vi "convertOldSetlist_toCluster_v5.vi"(0 "HW settings path":path=path "D:/My Documents/NIST (postdoc)/Labview/Data Acquisition/Hardware Control/Hardware/20121128_rbI_default_locked", 1 "Load pre 5.6 Globals?":bool, 5 "Procedure path":path=path "D:/My Documents/NIST (postdoc)/Labview/Data Acquisition/Hardware Control/procedures/201300927_Bzscan_Talbot", 7 "Version Selection":T4=enum."Load DDS 4.10", 11 "error in":errorcluster) -> (4 "Procedure Name":string, 10 "Save Cluster":T2={"Version"="", "Devices"=[], "Select Layout"=0, "Layout:Strings And Values []"=[], "User defined functions"="-- -------------------------------------------------------------------------------------------\n-- The following functions are part of the \"standard load\" of functions and should not be messed with\n-- They are here for reference only.\n-- Please add any user functions above this comment\n-- -------------------------------------------------------------------------------------------\n\n-- Creates a linear ramp from A to B\nfunction LineRamp(f, Initial, Final)\n    return (1-f)*Initial + f*Final;\nend\n\n-- Creates an exponential ramp from A to B\nfunction ExpRamp(t, a, b, tau)\n   return (b - a*exp(tMax / tau) + (a-b)*exp(t/tau))/ ( 1 - exp(tMax / tau) );\nend\n\n-- Creates a sinewave\nfunction SinRamp(t,Offset,A,Freq, Phase)\n    return Offset + A * sin(2*pi*Freq*t + Phase)\nend\n\n-- Creates a blackman pulse\nfunction Blackman(f, Offset, A)\n    return Offset +  A*sqrt(0.5*cos(3.1415*(2*f-1))+0.08*cos(2*pi*(2*f-1))+0.42);\nend\n\n-- Creates a half-gauss ramp\nfunction HalfGaussRamp(t, a, b, Width)\n    local y;\n    y = exp(-(tMax^2)/Width^2);\n    y = (a -  b*y)/(1-y)  +  ((b-a)/(1-y))*exp(-((t-tMax)^2)/Width^2);\n    return y;\nend\n\n-- Creates an \"O'Hara\" ramp from A to B, for dipole evaporation\nfunction EvapRamp(t, a, b, tau)\n   local y;\n  y = log(a/b) / log(1+tMax/tau);\n  y = a * (1+t/tau)^(-y);\n  return y;\nend\n", "VariableManager"=refnum} {"Select Layout" items=["Default"]}, 15 "error out":errorcluster)   [LabVIEW 2013]
uses:
  TypeDefs/Active procedure variables.ctl
  DeviceVIs/DDS/DDS.lvclass
  DeviceVIs/NI Card/NI Card.lvclass
  DeviceVIs/Novatech/Novatech.lvclass
  DeviceVIs/Pulseblaster/Pulseblaster.lvclass
  DeviceVIs/Device/Device.lvclass
  TypeDefs/PreviousVersionSelect.ctl
  TypeDefs/SaveCluster.ctl
  VariableManagerCodes/VariableManager/VariableManager.lvclass
  <vilib>/Utility/miscctls.llb/LVStringsAndValuesArrayTypeDef_I32.ctl
  VariableManagerCodes/API/VariableManagerAPI.lvlib
panel:
  in  "Tab Control":T1(tab)
  out "TempVariableManager":refnum<class "VariableManager.lvclass">
  out "Final PB Master Table":string[][](array[string])
  out "Final NI Device Table":string[][](array[string])
  out "Final Novatech Channel Table":string[][](array[string])
  out "Final DDS Table":string[][](array[string])
  out "DDS Object Array":refnum<class "DDS.lvclass">[](array[class])
  out "NI Card Array":refnum<class "NI Card.lvclass">[](array[class])
  in  "Master PulseBlaster":refnum<class "Pulseblaster.lvclass">
  out "Novatech Object Array":refnum<class "Novatech.lvclass">[](array[class])
  out "Slave PB Array":refnum<class "Pulseblaster.lvclass">[](array[class])
  out "Sequencing Info":T5(array[cluster])
  out "Static Variables":T6[](array[typedef])
  out "Devices":refnum<class "Device.lvclass">[](array[class])
  in  "Select Layout":i32(ring) items=["(On-the-fly)"=-2, "All"=-1, "Legacy"=0]
  out "User defined functions":string
  out "DDS Trig Lines":u16[](array[numeric])
  out "Novatech Trig Lines":u16[](array[numeric])
  out "NI Card Trig Lines":u16[](array[numeric])
  out "Version":string
  out "DDS Devices":T7(array[cluster])
  out "Slave Tables":T8
  out "Master Tables":T8
  out "Novatech Devices":T9(array[cluster])
  out "Novatech Ramps":T10(array[cluster])
  out "NI Cards":T11(array[cluster])
  out "SRS Ramps":T12(array[cluster])
  out "# of DO channels":i32
  out "# of AO channels":i32
  out "# DDS Devices":i32
  out "# Novatech devices":i32
  out "# NI Cards":i32
  out "Length of setlist (lines)":i32
  out "ColHdrs":string[](array[string])
  out "# of AI channels":i32
  # "Debugging:\n\nRight number of rows - YES\nMaster PB - Table = YES\nMaster PB - Hardware?\nDO - Table = Yes \nAO - Table = Yes\nNovatech - ???\nDDS - Table = Yes"
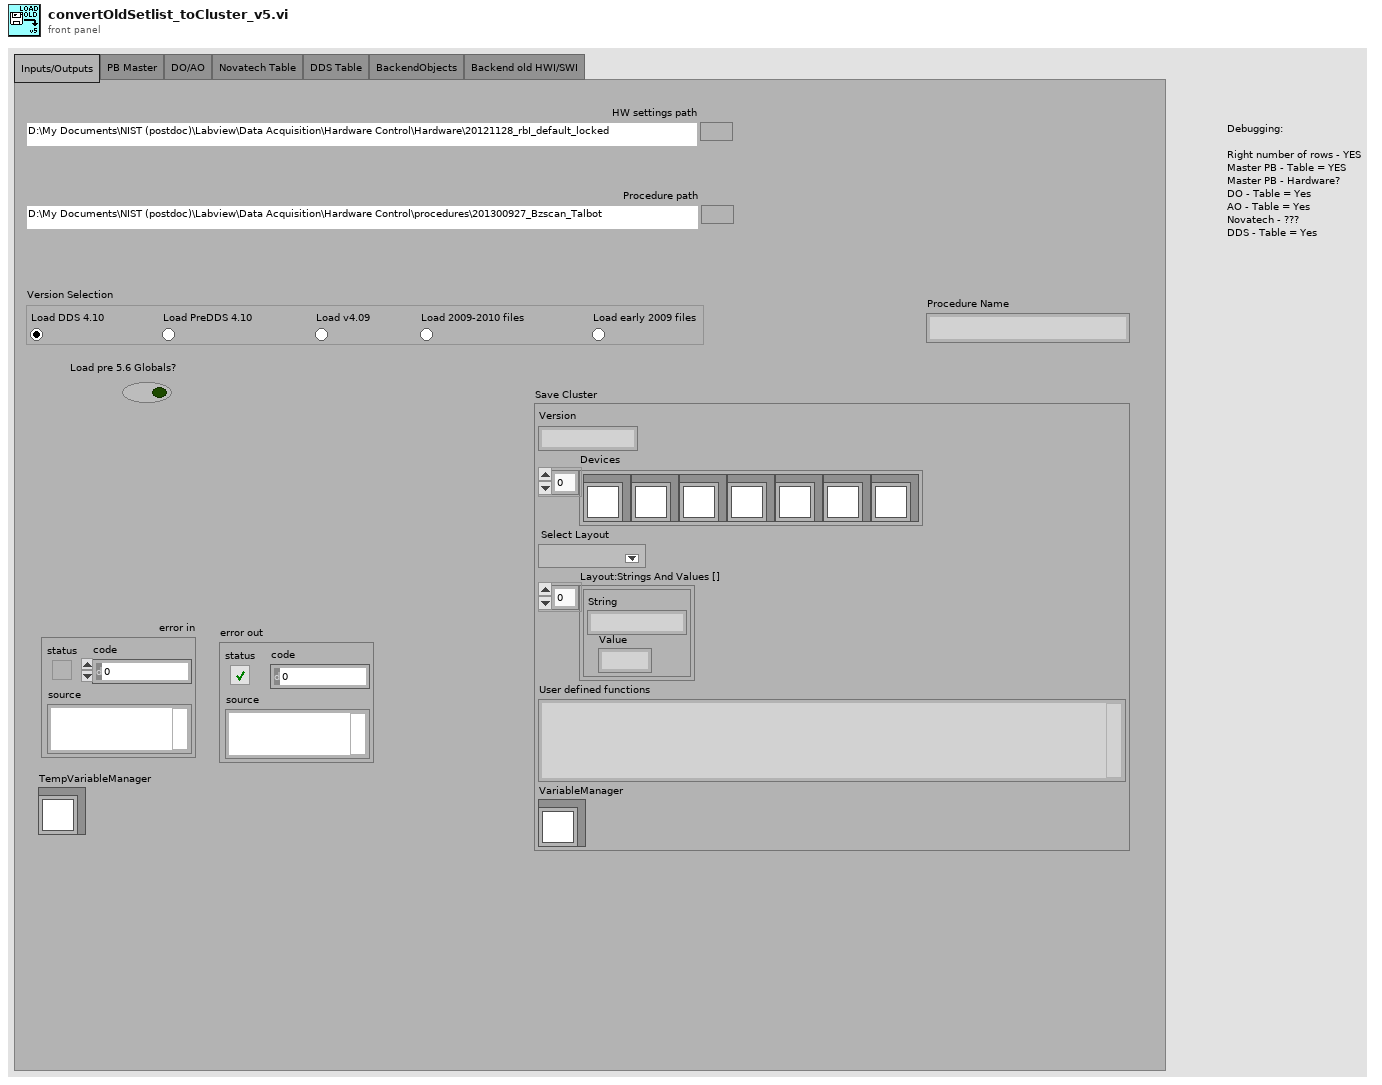
[diagram p1: front panel]
types:
  T1 = enum32{"Inputs/Outputs", "PB Master", "DO/AO", "Novatech Table", "DDS Table", "BackendObjects", "Backend old HWI/SWI"}
  T2 = typedef "SaveCluster.ctl" = cluster{"Version":string, "Devices":refnum<class "Device.lvclass">[], "Select Layout":i32, "Layout:Strings And Values []":T3, "User defined functions":string, "VariableManager":refnum<class "VariableManager.lvclass">}
  T3 = typedef "LVStringsAndValuesArrayTypeDef_I32.ctl" = cluster{"String":string, "Value":i32}[]
  T4 = typedef "PreviousVersionSelect.ctl" = enum32{"Load PreDDS 4.10", "Load early 2009 files", "Load 2009-2010 files", "Load DDS 4.10", "Load v4.09"}
  T5 = cluster{"Start":dbl, "End":dbl, "Sequenced Data":dbl[], "Inform\nIgor?":bool, "Computed Step Size":dbl, "Procedure Variable":string, "Default":dbl, "Steps":i32}[]
  T6 = typedef "Active procedure variables.ctl" = cluster{"Procedure variable":string, "Value":dbl}
  T7 = cluster{"PB Trigger Line":u16, "Sweeps":bool, "Channel Name":string, "Device Description":string, "PB trig / Sequence":bool, "Amp Lock":bool, "SetList Display":bool[], "FPGA Firmware Version":dbl}[]
  T8 = cluster{"Master Staging List":cluster{"Marker":string, "Mode":enum16{"Continue", "Ramp", "Loop", "EndLoop", "Halt"}, "Output Bits":bool[], "Delay (s)":string, "Ramp Step":dbl, "String":string, "Line Number":string}[], "Master DO Table":cluster{"Output Bits":bool[]}[], "Master AO Table":string[][], "Novatech Table":string[][], "DDS Table":string[][]}
  T9 = cluster{"PB Trigger Line":u16, "Serial Port":refnum<visa-resource-name>, "Channel Names":string[], "SetList Display":bool[][]}[]
  T10 = cluster{"Ramp Channels":cluster{"Time":string, "0 Freq. [MHz]":string, "0 Power [dBm]":string, "1 Freq. [MHz]":string, "1 Power [dBm]":string}[], "2 Freq. [MHz]":string, "2 Power [dBm]":string, "3 Freq. [MHz]":string, "3 Power [dBm]":string, "Serial Port":refnum<visa-resource-name>}[]
  T11 = cluster{"AO Channels":refnum<k21>[], "Trigger terminal":tag, "DO Channel":refnum<k21>, "AI Channels":refnum<k21>[], "PB Trigger Line":u16, "Trigger Mirror":tag, "DO lines":i32, "AO Channel Names":string[], "AI Channel Names":string[], "AI Pause Line":tag, "AI Sample Rate":dbl, "SetList Display":bool[]}[]
  T12 = cluster{"lattice ramp":cluster{"dt":string, "formula":string}[], "Output":cluster{"Time Values":dbl[], dbl[]}[], "SRS Selection":enum16{"1550 Vertical", "Bragg Agilent", "Bragg PTS", "Acc. Intensity"}}[]
  T13 = enum32{"Load PreDDS 4.10", "Load early 2009 files", "Load 2009-2010 files", "Load DDS 4.10", "Load v4.09"}
  T14 = cluster{"Master PB Staging List":cluster{"Output Bits":bool[], "Delay (s)":string, "String":string, "Halt?":bool}[], "Slave PB Staging List":cluster{"Output Bits":bool[], "Delay (s)":string, "String":string, "Halt?":bool}[], "Novatech Ramps":cluster{"Ramp Channels":cluster{"Time":string, "0 Freq. [MHz]":string, "0 Power [dBm]":string, "1 Freq. [MHz]":string, "1 Power [dBm]":string}[], "2 Freq. [MHz]":string, "2 Power [dBm]":string, "3 Freq. [MHz]":string, "3 Power [dBm]":string, "Serial Port":refnum<visa-resource-name>}[], "Sequencing Info":cluster{"Start":dbl, "End":dbl, "Sequenced Data":dbl[], "Inform\nIgor?":bool, "Computed Step Size":dbl, "Procedure Variable":string, "Default":dbl, "Steps":i32}[], "SRS Ramps":cluster{"lattice ramp":cluster{"dt":string, "formula":string}[], "Output":cluster{"Time Values":dbl[], dbl[]}[], "SRS Selection":enum16{"1550 Vertical", "Bragg Agilent", "Bragg PTS", "Acc. Intensity"}}[], "Master AO Ramp List":cluster{"Ramp index":u32, "Ramp time [s]":string, "Step size [s]":dbl, "Ramp Array":string[], "Output Bits":bool[]}[], "Slave AO Ramp List":cluster{"Ramp index":u32, "Ramp time [s]":string, "Step size [s]":dbl, "Ramp Array":string[], "Output Bits":bool[]}[], "Master Novatech Ramp List":cluster{"Ramp index":u32, "Ramp time [s]":string, "Step size [s]":dbl, "Data Array":string[]}[], "Static Variables":cluster{"Procedure variable":string, "Value":dbl}[], "DDS Ramp List":cluster{"Ramp index":u32, "Ramp time [s]":string, "Step size [s]":dbl, "Data Array":string[]}[]}
  T15 = cluster{"Master PB Staging List":cluster{"Output Bits":bool[], "Delay (s)":string, "String":string, "Halt?":bool}[], "Slave PB Staging List":cluster{"Output Bits":bool[], "Delay (s)":string, "String":string, "Halt?":bool}[], "Novatech Ramps":cluster{"Ramp Channels":cluster{"Time":string, "0 Freq. [MHz]":string, "0 Power [dBm]":string, "1 Freq. [MHz]":string, "1 Power [dBm]":string}[], "2 Freq. [MHz]":string, "2 Power [dBm]":string, "3 Freq. [MHz]":string, "3 Power [dBm]":string, "Serial Port":refnum<visa-resource-name>}[], "Sequencing Info":cluster{"Start":dbl, "End":dbl, "Sequenced Data":dbl[], "Inform\nIgor?":bool, "Computed Step Size":dbl, "Procedure Variable":string, "Default":dbl, "Steps":i32}[], "SRS Ramps":cluster{"lattice ramp":cluster{"dt":string, "formula":string}[], "Output":cluster{"Time Values":dbl[], dbl[]}[], "SRS Selection":enum16{"1550 Vertical", "Bragg Agilent", "Bragg PTS", "Acc. Intensity"}}[], "Master AO Ramp List":cluster{"Ramp index":u32, "Ramp time [s]":string, "Step size [s]":dbl, "Ramp Array":string[], "Output Bits":bool[]}[], "Slave AO Ramp List":cluster{"Ramp index":u32, "Ramp time [s]":string, "Step size [s]":dbl, "Ramp Array":string[], "Output Bits":bool[]}[], "Master Novatech Ramp List":cluster{"Ramp index":u32, "Ramp time [s]":string, "Step size [s]":dbl, "Data Array":string[]}[], "Static Variables":T6[], "DDS Ramp List":cluster{"Ramp index":u32, "Ramp time [s]":string, "Step size [s]":dbl, "Data Array":string[]}[]}
  T16 = cluster{"User defined functions":string, "Master AO Channels":cluster{"AO Channels":refnum<k21>[], "Trigger terminal":tag, "DO Channel":refnum<k21>, "AI Channels":refnum<k21>[], "PB Trigger Line":u16, "Trigger Mirror":tag, "DO lines":i32, "AO Channel Names":string[], "AI Channel Names":string[], "AI Pause Line":tag, "AI Sample Rate":dbl, "SetList Display":bool[]}[], "Novatech Devices":cluster{"PB Trigger Line":u16, "Serial Port":refnum<visa-resource-name>, "Channel Names":string[], "SetList Display":bool[][]}[], "DDS Devices":cluster{"PB Trigger Line":u16, "Sweeps":bool, "Channel Name":string, "Device Description":string, "PB trig / Sequence":bool, "Amp Lock":bool, "SetList Display":bool[], "FPGA Firmware Version":dbl}[]}
  T17 = cluster{"Output Bits":bool[], "Delay (s)":string, "String":string, "Halt?":bool}[]
  T18 = cluster{"Ramp index":u32, "Ramp time [s]":string, "Step size [s]":dbl, "Ramp Array":string[], "Output Bits":bool[]}[]
  T19 = cluster{"Ramp index":u32, "Ramp time [s]":string, "Step size [s]":dbl, "Data Array":string[]}[]
  T20 = cluster{"Marker":string, "Mode":enum16{"Continue", "Ramp", "Loop", "EndLoop", "Halt"}, "Output Bits":bool[], "Delay (s)":string, "Ramp Step":dbl, "String":string, "Line Number":string}[]
  T21 = enum16{"Continue", "Ramp", "Loop", "EndLoop", "Halt"}
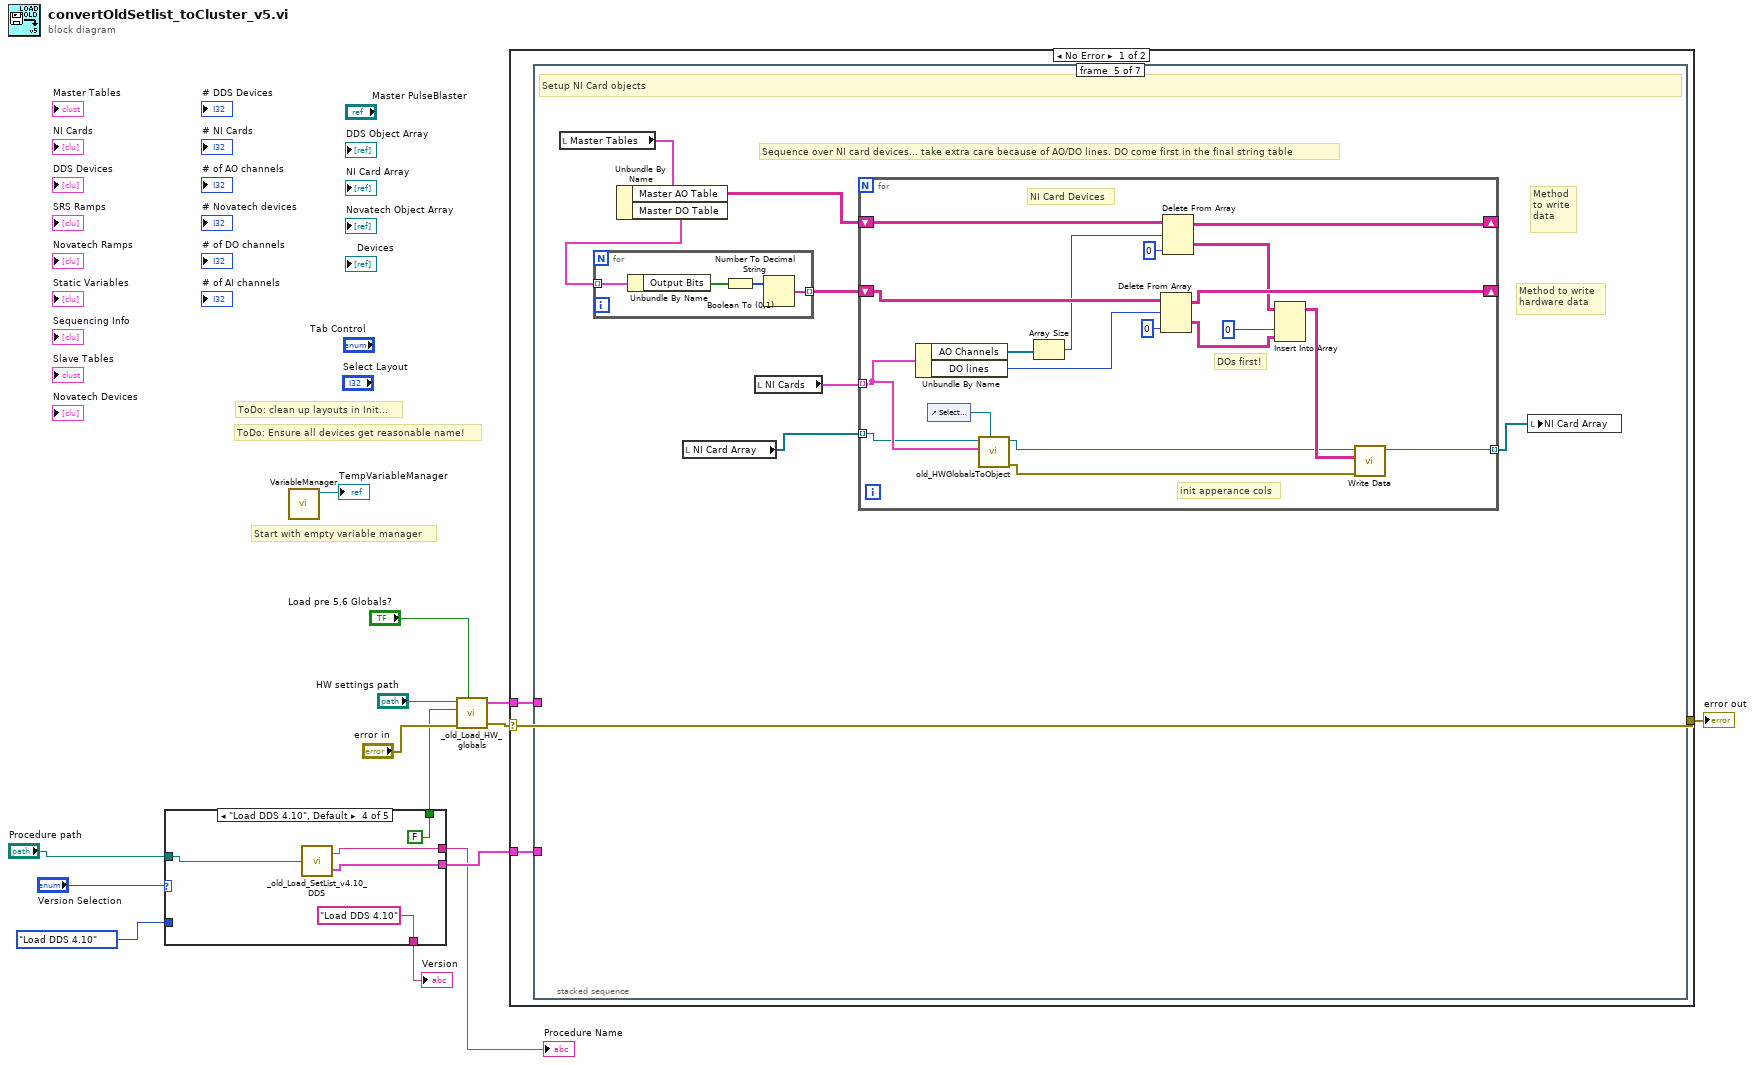
[diagram p0: block diagram]
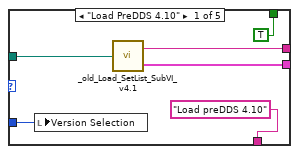
[diagram p2: hidden frame]
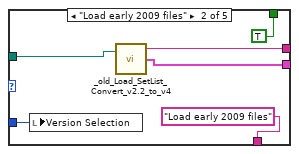
[diagram p3: hidden frame]
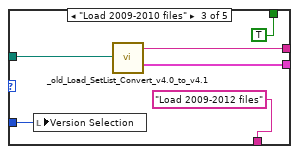
[diagram p4: hidden frame]
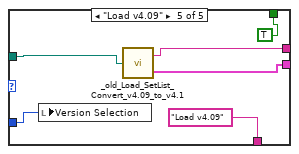
[diagram p5: hidden frame]
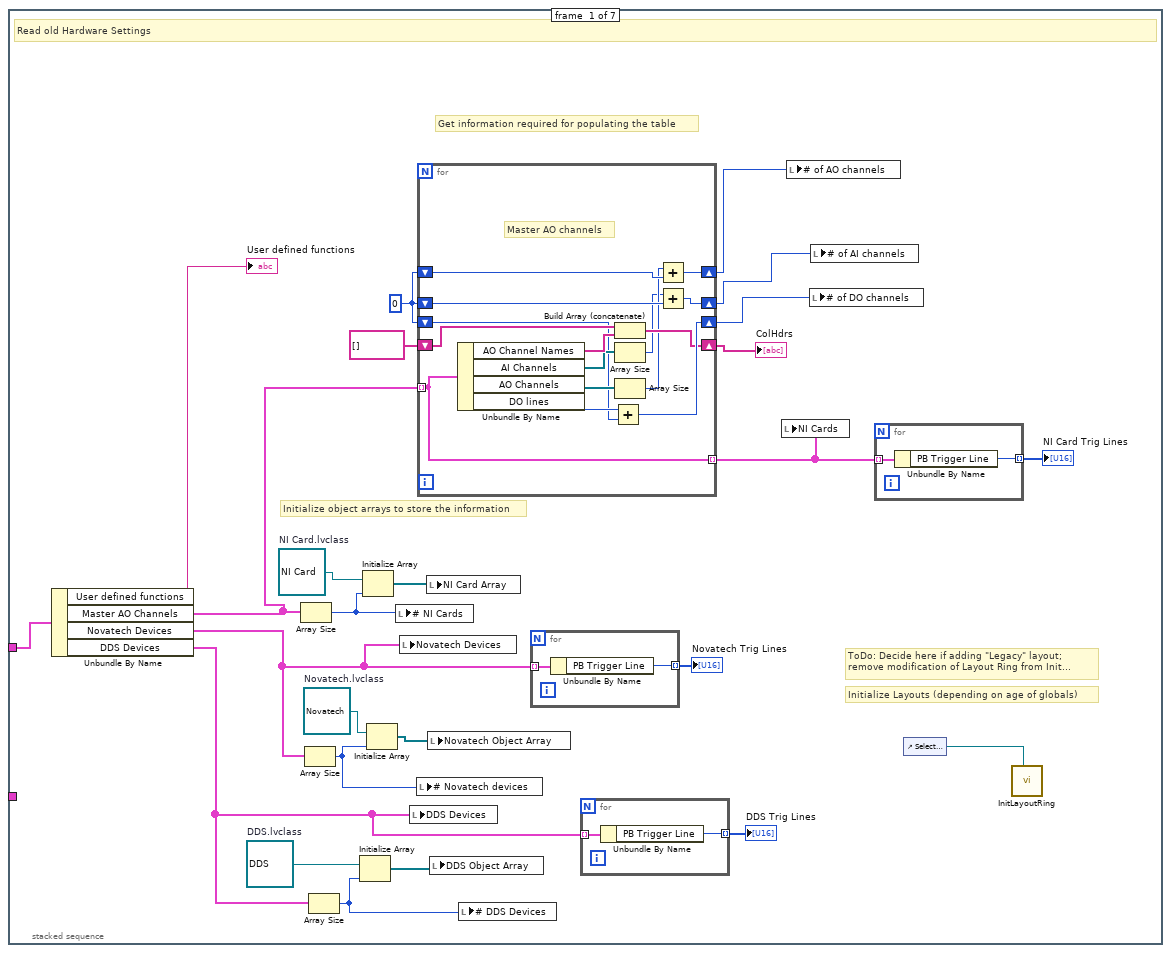
[diagram p6: hidden frame]
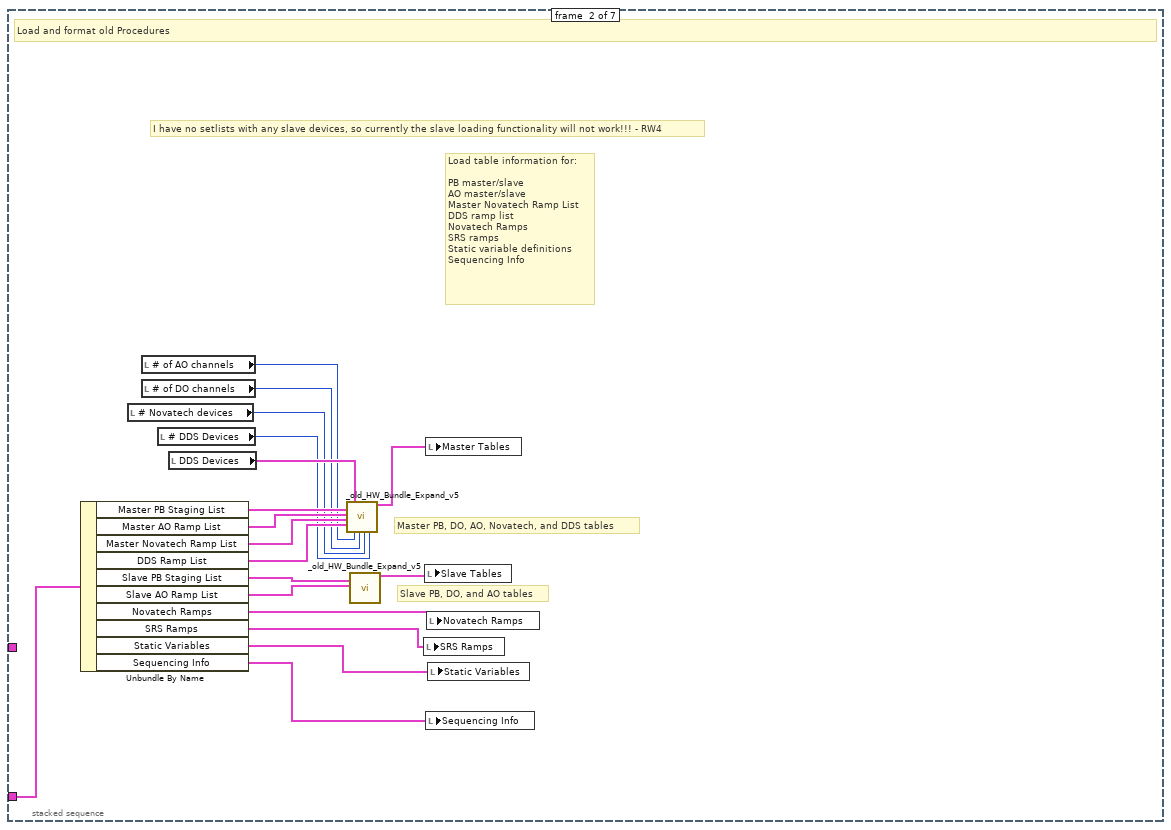
[diagram p7: hidden frame]
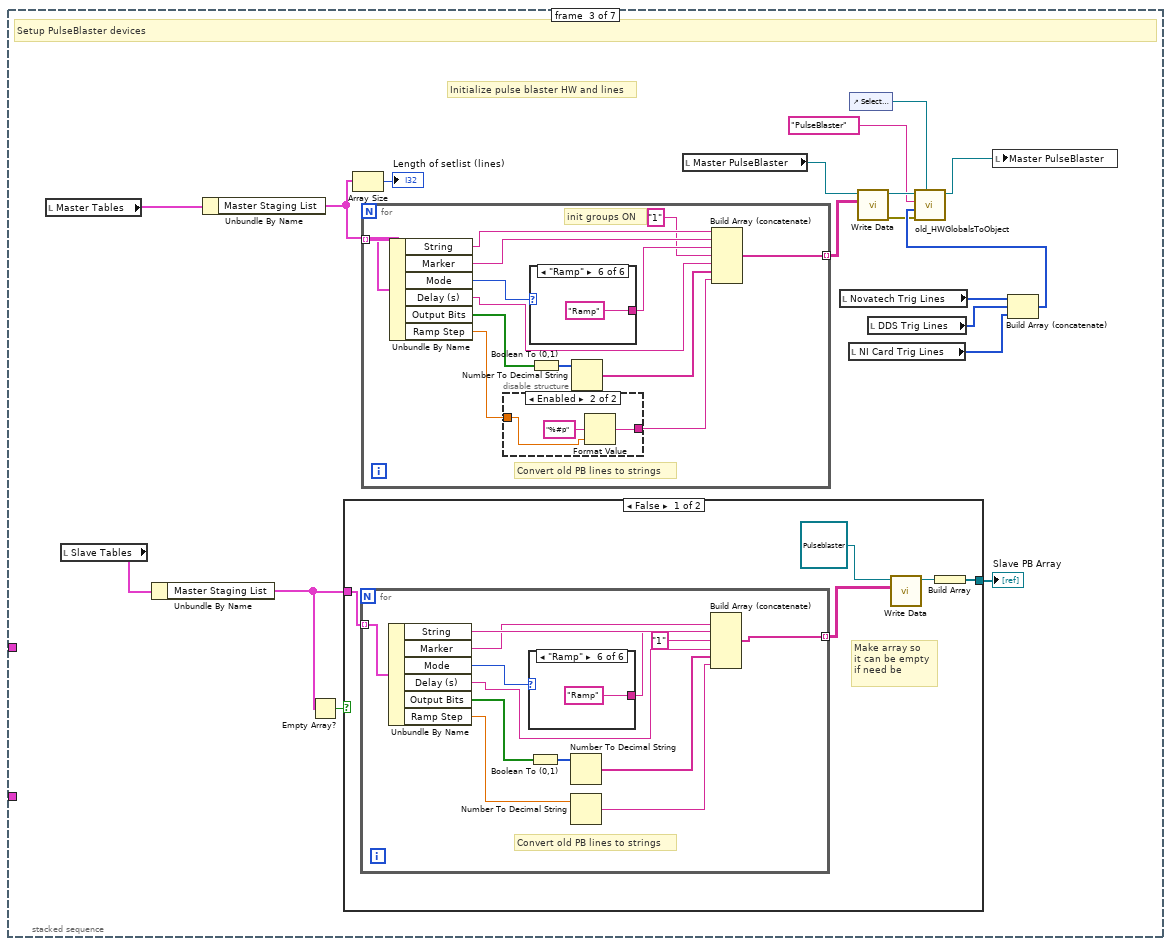
[diagram p8: hidden frame]
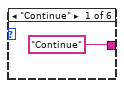
[diagram p9: hidden frame]
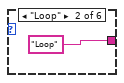
[diagram p10: hidden frame]
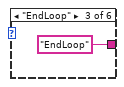
[diagram p11: hidden frame]
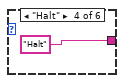
[diagram p12: hidden frame]
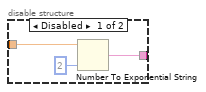
[diagram p15: hidden frame]
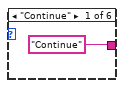
[diagram p16: hidden frame]
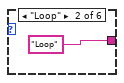
[diagram p17: hidden frame]
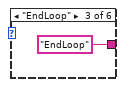
[diagram p18: hidden frame]
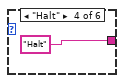
[diagram p19: hidden frame]
diagram:
  # "Start with empty variable manager"
  # "ToDo: Ensure all devices get reasonable name!"
  # "ToDo: clean up layouts in Init..."
  n1 = case shown="\"Load DDS 4.10\", Default" "Version Selection" {
    tunnel: [w20 w25 w32 w36 w40] -> w6
    tunnel: "Procedure path" -> [w19 w26 w30 w37 w41]
    tunnel: [w18 w24 w31 w35 w39] -> w7
    tunnel: T13."Load DDS 4.10" ("Version Selection") -> [w17 w23 w29 _ w43]
    tunnel: [TRUE TRUE TRUE FALSE TRUE] -> w4
    tunnel: ["Load preDDS 4.10" "Load early 2009 files" "Load 2009-2012 files" "Load DDS 4.10" "Load v4.09"] -> w2
    frame "Load PreDDS 4.10" {
      n2 = local write "Version Selection"(w17) -> ()
      n3 = call "_old_Load_SetList_SubVI_v4.1.vi"("Path"=w19) -> ("Procedure Name"=w20:string, "Paramaters"=w18:T14)
    }
    frame "Load early 2009 files" {
      n4 = local write "Version Selection"(w23) -> ()
      n5 = call "_old_Load_SetList_Convert_v2.2_to_v4.vi"("Path"=w26) -> ("Procedure Name"=w25:string, "Paramaters"=w24:T14)  [unwired: 1 in, 1 out]
    }
    frame "Load 2009-2010 files" {
      n6 = local write "Version Selection"(w29) -> ()
      n7 = call "_old_Load_SetList_Convert_v4.0_to_v4.1.vi"("Path"=w30) -> ("Procedure Name"=w32:string, "Paramaters"=w31:T14)
    }
    frame "Load DDS 4.10", Default {
      n8 = call "_old_Load_SetList_v4.10_DDS.vi"("Path"=w37) -> ("Procedure Name"=w36:string, "Paramaters"=w35:T15)
    }
    frame "Load v4.09" {
      n9 = local write "Version Selection"(w43) -> ()
      n10 = call "_old_Load_SetList_Convert_v4.09_to_v4.1.vi"("Path"=w41) -> ("Procedure Name"=w40:string, "Paramaters"=w39:T14)
    }
  }
  "Procedure Name" <- w6
  "Version" <- w2
  n11 = call "VariableManager.vi"() -> ("VariableManager"=→"TempVariableManager":refnum<class "VariableManager.lvclass">)  [unwired: 11 in]
  n12 = call "_old_Load_HW_globals.vi"("HW settings path"="HW settings path", "Load pre 5.6 Globals?"="Load pre 5.6 Globals?", "Pre 4.1 HWGlobals?"=w4, "error in"="error in") -> ("Loaded Procedure Data"=w14:T16, "error out"=w3:errorcluster)  [unwired: 2 in, 1 out]
  n13 = case shown="No Error" w3 {
    selector: w3 -> [w44 w315]
    tunnel: w7 -> [w45 _]
    tunnel: w14 -> [w46 _]
    tunnel: [w44 w315] -> w10
    frame No Error {
      n14 = stacked-sequence {
        tunnel: w46 -> [w71 _ _ _ _ _ _]
        tunnel: w45 -> [_ w110 _ _ _ _ _]
        frame #0 {
          w61 = refnum<class "Novatech.lvclass"> refnum  # Novatech.lvclass
          w62 = refnum<class "NI Card.lvclass"> refnum  # NI Card.lvclass
          w63 = refnum<class "DDS.lvclass"> refnum  # DDS.lvclass
          w68 = 0
          # "ToDo: Decide here if adding \"Legacy\" layout;\nremove modification of Layout Ring from Init..."
          # "Initialize Layouts (depending on age of globals)"
          # "Initialize object arrays to store the information"
          # "Get information required for populating the table"
          # "Read old Hardware Settings"
          n15 = Unbundle By Name(w71) -> ("User defined functions"=→"User defined functions":string, "Master AO Channels"=w67:T11, "Novatech Devices"=w54:T9, "DDS Devices"=w52:T7)
          n16 = Array Size(array=w67) -> (size(s)=w60:i32)
          n17 = Array Size(array=w54) -> (size(s)=w57:i32)
          n18 = Array Size(array=w52) -> (size(s)=w58:i32)
          n19 = Initialize Array(w63, w58) -> (w47:refnum<class "DDS.lvclass">[])
          n20 = Initialize Array(w62, w60) -> (w49:refnum<class "NI Card.lvclass">[])
          n21 = Initialize Array(w61, w57) -> (w48:refnum<class "Novatech.lvclass">[])
          n22 = local write "# NI Cards"(w60) -> ()
          n23 = local write "Novatech Devices"(w54) -> ()
          n24 = local write "DDS Devices"(w52) -> ()
          n25 = local write "# Novatech devices"(w57) -> ()
          n26 = for {
            tunnel: w67 -> [w81] mode=indexing
            shift-right: [w90] -> w65
            shift-left: w68 -> [w79]
            shift-right: [w89] -> w64
            shift-left: w68 -> [w91]
            shift-right: [w88] -> w66
            shift-left: w68 -> [w92]
            shift-right: [w84] -> w69
            shift-left: string[] [] ("initialized array") -> [w85]
            tunnel: [w81] -> w56 mode=indexing
            # "Master AO channels"
            n27 = Unbundle By Name(w81) -> ("AO Channel Names"=w86:string[], "AI Channels"=w83:refnum<k21>[], "AO Channels"=w82:refnum<k21>[], "DO lines"=w87:i32)
            n28 = Add(x=w87, y=w79) -> (x+y=w90:i32)
            n29 = Build Array (concatenate)(w85, w86) -> (w84:string[])
            n30 = Array Size(array=w83) -> (size(s)=w78:i32)
            n31 = Array Size(array=w82) -> (size(s)=w80:i32)
            n32 = Add(x=w80, y=w92) -> (x+y=w88:i32)
            n33 = Add(x=w78, y=w91) -> (x+y=w89:i32)
          }
          "ColHdrs" <- w69
          n34 = local write "NI Card Array"(w49) -> ()
          n35 = local write "Novatech Object Array"(w48) -> ()
          n36 = local write "DDS Object Array"(w47) -> ()
          n37 = local write "# DDS Devices"(w58) -> ()
          n38 = for {
            tunnel: w54 -> [w75] mode=indexing
            tunnel: [w74] -> w53 mode=indexing
            n39 = Unbundle By Name(w75) -> ("PB Trigger Line"=w74:u16)
          }
          "Novatech Trig Lines" <- w53
          n40 = for {
            tunnel: w52 -> [w73] mode=indexing
            tunnel: [w72] -> w51 mode=indexing
            n41 = Unbundle By Name(w73) -> ("PB Trigger Line"=w72:u16)
          }
          "DDS Trig Lines" <- w51
          n42 = local write "NI Cards"(w56) -> ()
          n43 = local write "# of AO channels"(w66) -> ()
          n44 = local write "# of DO channels"(w65) -> ()
          n45 = local write "# of AI channels"(w64) -> ()
          n46 = for {
            tunnel: w56 -> [w77] mode=indexing
            tunnel: [w76] -> w55 mode=indexing
            n47 = Unbundle By Name(w77) -> ("PB Trigger Line"=w76:u16)
          }
          "NI Card Trig Lines" <- w55
          n48 = control-ref of="Select Layout"() -> (w50:refnum<vi>)
          n49 = call "InitLayoutRing.vi"("Layouts Ring Refnum"=w50) -> ()  [unwired: 10 in, 1 out]
        }
        frame #1 {
          # "I have no setlists with any slave devices, so currently the slave loading functionality will not work!!! - RW4"
          # "Load table information for:\n\nPB master/slave\nAO master/slave\nMaster Novatech Ramp List\nDDS ramp list\nNovatech Ramps\nSRS ramps\nStatic variable definitions\nSequencing Info"
          # "Slave PB, DO, and AO tables"
          # "Master PB, DO, AO, Novatech, and DDS tables"
          # "Load and format old Procedures"
          n50 = Unbundle By Name(w110) -> ("Master PB Staging List"=w109:T17, "Master AO Ramp List"=w108:T18, "Master Novatech Ramp List"=w107:T19, "DDS Ramp List"=w106:T19, "Slave PB Staging List"=w104:T17, "Slave AO Ramp List"=w103:T18, "Novatech Ramps"=w101:T10, "SRS Ramps"=w102:T12, "Static Variables"=w99:T6[], "Sequencing Info"=w100:T5)
          n51 = local read "# Novatech devices"() -> (w94:i32)
          n52 = local read "# of AO channels"() -> (w96:i32)
          n53 = local read "# of DO channels"() -> (w95:i32)
          n54 = local read "# DDS Devices"() -> (w93:i32)
          n55 = local read "DDS Devices"() -> (w105:T7)
          n56 = call "_old_HW_Bundle_Expand_v5.vi"("PB Staging List"=w109, "AO Ramp List"=w108, "Novatech Ramp List"=w107, "DDS Ramp List"=w106, "DDS Devices"=w105, "Number of AO channels"=w96, "Number of DO channels"=w95, "Number of Novatech channels"=w94, "Number of DDS channels"=w93) -> ("Master Tables"=w98:T8)  [unwired: 10 in]
          n57 = call "_old_HW_Bundle_Expand_v5.vi"("PB Staging List"=w104, "AO Ramp List"=w103) -> ("Master Tables"=w97:T8)  [unwired: 17 in]
          n58 = local write "SRS Ramps"(w102) -> ()
          n59 = local write "Slave Tables"(w97) -> ()
          n60 = local write "Master Tables"(w98) -> ()
          n61 = local write "Sequencing Info"(w100) -> ()
          n62 = local write "Novatech Ramps"(w101) -> ()
          n63 = local write "Static Variables"(w99) -> ()
        }
        frame #2 {
          # "Initialize pulse blaster HW and lines"
          # "Setup PulseBlaster devices"
          n64 = local read "Master Tables"() -> (w128:T8)
          n65 = local read "Slave Tables"() -> (w123:T8)
          n66 = Unbundle By Name(w123) -> ("Master Staging List"=w122:T20)
          n67 = Unbundle By Name(w128) -> ("Master Staging List"=w126:T20)
          n68 = Empty Array?(array=w122) -> (empty?=w121:bool)
          n69 = case shown="False" w121 {
            tunnel: w122 -> [w132 _]
            tunnel: [w130 _] -> w111
            frame False {
              # "Make array so\nit can be empty\nif need be"
              n70 = for {
                tunnel: w132 -> [w146] mode=indexing
                tunnel: [w138] -> w133 mode=indexing
                # "Convert old PB lines to strings"
                n71 = Unbundle By Name(w146) -> ("String"=w145:string, "Marker"=w144:string, "Mode"=w143:T21, "Delay (s)"=w135:string, "Output Bits"=w140:bool[], "Ramp Step"=w141:dbl)
                n72 = case shown="\"Ramp\"" w143 {
                  tunnel: ["Continue" "Loop" "EndLoop" "Halt" _ "Ramp"] -> w142
                  frame "Continue" {
                  }
                  frame "Loop" {
                  }
                  frame "EndLoop" {
                  }
                  frame "Halt" {
                  }
                  frame Default {
                  }
                  frame "Ramp" {
                  }
                }
                n73 = Boolean To (0,1)(Boolean=w140) -> (0, 1=w139:i16[])
                n74 = Number To Decimal String(number=w139) -> (decimal integer string=w136:string[])  [unwired: 1 in]
                n75 = Number To Decimal String(number=w141) -> (decimal integer string=w137:string)  [unwired: 1 in]
                n76 = Build Array (concatenate)(w145, w144, w142, "1" ("element"), w135, w136, w137) -> (w138:string[])
              }
              n77 = call-dynamic "Write Data.vi"("Data"=w133, "Device in"=refnum<class "Pulseblaster.lvclass"> refnum ("Master PulseBlaster")) -> ("Device Out"=w131:refnum<class "Pulseblaster.lvclass">)  [unwired: 8 in, 1 out]
              n78 = Build Array(w131) -> (w130:refnum<class "Pulseblaster.lvclass">[])
            }
            frame True {
              # "No Slave PB"
            }
          }
          "Slave PB Array" <- w111
          n79 = Array Size(array=w126) -> (size(s)=→"Length of setlist (lines)":i32)
          n80 = for {
            tunnel: w126 -> [w164] mode=indexing
            tunnel: [w157] -> w125 mode=indexing
            # "init groups ON"
            # "Convert old PB lines to strings"
            n81 = Unbundle By Name(w164) -> ("String"=w163:string, "Marker"=w162:string, "Mode"=w161:T21, "Delay (s)"=w155:string, "Output Bits"=w159:bool[], "Ramp Step"=w152:dbl)
            n82 = disable-structure shown="Enabled" {
              disable-tunnel: [w167 w169] -> w153
              disable-tunnel: w152 -> [w166 w168]
              frame Disabled {
                n83 = Number To Exponential String(number=w166, precision (6)=i16 2) -> (E-format string=w167:string)  [unwired: 2 in]
              }
              frame Enabled {
                n84 = Format Value(format string="%#p", value (0)=w168) -> (output string=w169:string)  [unwired: 1 in]
              }
            }
            n85 = case shown="\"Ramp\"" w161 {
              tunnel: ["Continue" "Loop" "EndLoop" "Halt" _ "Ramp"] -> w160
              frame "Continue" {
              }
              frame "Loop" {
              }
              frame "EndLoop" {
              }
              frame "Halt" {
              }
              frame Default {
              }
              frame "Ramp" {
              }
            }
            n86 = Boolean To (0,1)(Boolean=w159) -> (0, 1=w158:i16[])
            n87 = Number To Decimal String(number=w158) -> (decimal integer string=w156:string[])  [unwired: 1 in]
            n88 = Build Array (concatenate)(w163, w162, w160, "1" ("element"), w155, w156, w153) -> (w157:string[])
          }
          n89 = local read "Master PulseBlaster"() -> (w124:refnum<class "Pulseblaster.lvclass">)
          n90 = local read "Novatech Trig Lines"() -> (w117:u16[])
          n91 = local read "NI Card Trig Lines"() -> (w115:u16[])
          n92 = control-ref of="Select Layout"() -> (w112:refnum<vi>)
          n93 = call-dynamic "Write Data.vi"("Data"=w125, "Device in"=w124) -> ("error out"=w113:errorcluster, "Device Out"=w120:refnum<class "Pulseblaster.lvclass">)  [unwired: 8 in]
          n94 = local read "DDS Trig Lines"() -> (w116:u16[])
          n95 = Build Array (concatenate)(w117, w116, w115) -> (w114:u16[])
          n96 = call "old_HWGlobalsToObject.vi"("Select Layout"=w112, "error in (no error)"=w113, "Trigger Lines"=w114, "Name"="PulseBlaster", "Pulseblaster in"=w120) -> ("Pulseblaster out"=w119:refnum<class "Pulseblaster.lvclass">)  [unwired: 5 in, 1 out]
          n97 = local write "Master PulseBlaster"(w119) -> ()
        }
        frame #3 {
          # "Sequence over old master tables\nGrab individual software image table that corresponds to each device"
          # "Setup Novatech and DDS devices"
          n98 = local read "Master Tables"() -> (w180:T8)
          n99 = local read "Novatech Object Array"() -> (w178:refnum<class "Novatech.lvclass">[])
          n100 = Unbundle By Name(w180) -> ("DDS Table"=w183:string[][])
          n101 = Unbundle By Name(w180) -> ("Novatech Table"=w182:string[][])
          n102 = local read "Novatech Devices"() -> (w181:T9)
          n103 = local read "DDS Object Array"() -> (w179:refnum<class "DDS.lvclass">[])
          n104 = local read "DDS Devices"() -> (w184:T7)
          n105 = for {
            tunnel: w179 -> [w201] mode=indexing
            tunnel: w184 -> [w199] mode=indexing
            shift-right: [w202] -> _
            shift-left: w183 -> [w206]
            tunnel: [w203] -> w176 mode=indexing
            # "DDS Devices"
            n106 = control-ref of="Select Layout"() -> (w197:refnum<vi>)
            n107 = Unbundle By Name(w199) -> ("Sweeps"=w207:bool)
            n108 = call "old_HWGlobalsToObject.vi"("Select Layout"=w197, "DDS Device"=w199, "DDS in"=w201) -> ("error out"=w196:errorcluster, "DDS out"=w200:refnum<class "DDS.lvclass">)  [unwired: 7 in]
            n109 = case shown="False" w207 {
              tunnel: [3 5] -> w204
              frame False {
              }
              frame True {
              }
            }
            n110 = Delete From Array(array=w206, length=w204, index (col)=0 ("disabled index (col)")) -> (deleted portion=w198:string[][], array with subset deleted=w202:string[][])  [unwired: 1 in]
            n111 = call-dynamic "Write Data.vi"("error in (no error)"=w196, "Data"=w198, "Device in"=w200) -> ("Device Out"=w203:refnum<class "DDS.lvclass">)  [unwired: 7 in, 1 out]
          }
          n112 = for {
            tunnel: w178 -> [w189] mode=indexing
            tunnel: w181 -> [w187] mode=indexing
            shift-right: [w194] -> _
            shift-left: w182 -> [w195]
            tunnel: [w191] -> w177 mode=indexing
            # "Novatech Devices"
            n113 = control-ref of="Select Layout"() -> (w186:refnum<vi>)
            n114 = Delete From Array(array=w195, length=12, index (col)=0 ("disabled index (col)")) -> (deleted portion=w190:string[][], array with subset deleted=w194:string[][])  [unwired: 1 in]
            n115 = call "old_HWGlobalsToObject.vi"("Select Layout"=w186, "Novatech Channel"=w187, "Novatech in"=w189) -> ("error out"=w185:errorcluster, "Novatech out"=w188:refnum<class "Novatech.lvclass">)  [unwired: 7 in]
            n116 = call-dynamic "Write Data.vi"("error in (no error)"=w185, "Data"=w190, "Device in"=w188) -> ("Device Out"=w191:refnum<class "Novatech.lvclass">)  [unwired: 7 in, 1 out]
          }
          n117 = local write "Novatech Object Array"(w177) -> ()
          n118 = local write "DDS Object Array"(w176) -> ()
        }
        frame #4 {
          # "Sequence over NI card devices... take extra care because of AO/DO lines. DO come first in the final string table"
          # "Method to write\nhardware data"
          # "Method\nto write\ndata"
          # "Setup NI Card objects"
          n119 = local read "Master Tables"() -> (w215:T8)
          n120 = Unbundle By Name(w215) -> ("Master AO Table"=w214:string[][], "Master DO Table"=w213:cluster{"Output Bits":bool[]}[])
          n121 = for {
            tunnel: [w218] -> w212 mode=indexing
            tunnel: w213 -> [w217] mode=indexing
            n122 = Unbundle By Name(w217) -> ("Output Bits"=w220:bool[])
            n123 = Boolean To (0,1)(Boolean=w220) -> (0, 1=w219:i16[])
            n124 = Number To Decimal String(number=w219) -> (decimal integer string=w218:string[])  [unwired: 1 in]
          }
          n125 = local read "NI Card Array"() -> (w211:refnum<class "NI Card.lvclass">[])
          n126 = local read "NI Cards"() -> (w216:T11)
          n127 = for {
            shift-right: [w233] -> _
            shift-left: w214 -> [w239]
            tunnel: w216 -> [w229] mode=indexing
            shift-right: [w234] -> _
            shift-left: w212 -> [w236]
            tunnel: [w230] -> w210 mode=indexing
            tunnel: w211 -> [w228] mode=indexing
            # "init apperance cols"
            # "DOs first!"
            # "NI Card Devices"
            n128 = Unbundle By Name(w229) -> ("AO Channels"=w235:refnum<k21>[], "DO lines"=w224:i32)
            n129 = control-ref of="Select Layout"() -> (w221:refnum<vi>)
            n130 = call "old_HWGlobalsToObject.vi"("Select Layout"=w221, "Master AO Channel"=w229, "NI Card in"=w228) -> ("error out"=w222:errorcluster, "NI Card out"=w223:refnum<class "NI Card.lvclass">)  [unwired: 7 in]
            n131 = Array Size(array=w235) -> (size(s)=w225:i32)
            n132 = Delete From Array(array=w236, length=w224, index (col)=0 ("disabled index (col)")) -> (deleted portion=w226:string[][], array with subset deleted=w234:string[][])  [unwired: 1 in]
            n133 = Delete From Array(array=w239, length=w225, index (col)=0 ("disabled index (col)")) -> (deleted portion=w227:string[][], array with subset deleted=w233:string[][])  [unwired: 1 in]
            n134 = Insert Into Array(array=w227, index (col)=0 ("disabled index (col)"), new element=w226) -> (w231:string[][])  [unwired: 1 in]
            n135 = call-dynamic "Write Data.vi"("error in (no error)"=w222, "Data"=w231, "Device in"=w223) -> ("Device Out"=w230:refnum<class "NI Card.lvclass">)  [unwired: 7 in, 1 out]
          }
          n136 = local write "NI Card Array"(w210) -> ()
        }
        frame #5 {
          # "Store final device object array"
          # "Build device array; Device tables for testing"
          n137 = local read "Master PulseBlaster"() -> (w254:refnum<class "Pulseblaster.lvclass">)
          n138 = local read "Novatech Object Array"() -> (w240:refnum<class "Novatech.lvclass">[])
          n139 = local read "DDS Object Array"() -> (w242:refnum<class "DDS.lvclass">[])
          n140 = local read "NI Card Array"() -> (w241:refnum<class "NI Card.lvclass">[])
          n141 = Build Array(w254) -> (w253:refnum<class "Pulseblaster.lvclass">[])
          n142 = Insert Into Array(array=refnum<class "Device.lvclass">[] [] ("Devices 2"), new element #1=w253, new element #2=w241, new element #3=w240, new element #4=w242) -> (w243:refnum<class "Device.lvclass">[])  [unwired: 1 in]
          n143 = local write "Devices"(w243) -> ()
          n144 = for {
            tunnel: w253 -> [w266] mode=indexing
            tunnel: [w264] -> w252 mode=concatenating
            # "PB Master"
            n145 = call-dynamic "Get Data.vi"("Device in"=w266) -> ("Table Indicator"=w265:string[][])  [unwired: 7 in, 2 out]
            n146 = Transpose 2D Array(2D array=w265) -> (transposed array=w264:string[][])
          }
          n147 = for {
            tunnel: [w258] -> w247 mode=concatenating
            tunnel: w240 -> [w260] mode=indexing
            # "Novatech"
            n148 = call-dynamic "Get Data.vi"("Device in"=w260) -> ("Table Indicator"=w259:string[][])  [unwired: 7 in, 2 out]
            n149 = Transpose 2D Array(2D array=w259) -> (transposed array=w258:string[][])
          }
          n150 = for {
            tunnel: [w261] -> w249 mode=concatenating
            tunnel: w241 -> [w263] mode=indexing
            # "NI Card"
            n151 = call-dynamic "Get Data.vi"("Device in"=w263) -> ("Table Indicator"=w262:string[][])  [unwired: 7 in, 2 out]
            n152 = Transpose 2D Array(2D array=w262) -> (transposed array=w261:string[][])
          }
          n153 = for {
            tunnel: [w255] -> w245 mode=concatenating
            tunnel: w242 -> [w257] mode=indexing
            # "DDS"
            n154 = call-dynamic "Get Data.vi"("Device in"=w257) -> ("Table Indicator"=w256:string[][])  [unwired: 7 in, 2 out]
            n155 = Transpose 2D Array(2D array=w256) -> (transposed array=w255:string[][])
          }
          n156 = Transpose 2D Array(2D array=w245) -> (transposed array=→"Final DDS Table":string[][])
          n157 = Transpose 2D Array(2D array=w247) -> (transposed array=→"Final Novatech Channel Table":string[][])
          n158 = Transpose 2D Array(2D array=w249) -> (transposed array=→"Final NI Device Table":string[][])
          n159 = Transpose 2D Array(2D array=w252) -> (transposed array=→"Final PB Master Table":string[][])
        }
        frame #6 {
          # "Build \"Save Cluster\": Re-shape variables and bundle devices, layout..."
          n160 = flat-sequence {
            tunnel: [w278] -> w275
            tunnel: w275 -> [w314]
            tunnel: [w313] -> w274
            frame #0 {
              w282 = "idx"
              n161 = local read "Sequencing Info"() -> (w284:T5)
              n162 = local read "Static Variables"() -> (w280:T6[])
              n163 = control-ref of="TempVariableManager"() -> (w276:refnum<vi>)
              n164 = for {
                tunnel: w280 -> [w290] mode=indexing
                tunnel: w276 -> [w287]
                n165 = Unbundle(w290) -> ("Procedure variable"=w289:string, "Value"=w288:dbl)
                n166 = call "Variable.vi"("VariableName"=w289, "DefaultValue"=w288) -> ("Variable"=w286:refnum<class "Variable.lvclass">)  [unwired: 9 in]
                n167 = call "VariableWrite.vi"("Variable"=w286, "VariableManagerRef in"=w287) -> ("error out"=w285:errorcluster)  [unwired: 8 in, 1 out]
                n168 = call "DisplayMessageAsync.vi"("error in (no error)"=w285) -> ()  [unwired: 11 in]
              }
              n169 = for {
                tunnel: w284 -> [w304] mode=indexing
                tunnel: w282 -> [w303]
                tunnel: [w302] -> w283
                tunnel: w276 -> [w292]
                n170 = Unbundle By Name(w304) -> ("Start"=w301:dbl, "End"=w300:dbl, "Inform\nIgor?"=w295:bool, "Procedure Variable"=w299:string, "Default"=w298:dbl, "Steps"=w302:i32)  [unwired: 2 out]
                n171 = Not Equal?(x=w301, y=w300) -> (x != y?=w293:bool)
                n172 = case shown="True" w293 {
                  selector: w293 -> [w306 w307]
                  tunnel: w303 -> [_ w311]
                  tunnel: w301 -> [_ w310]
                  tunnel: w300 -> [_ w309]
                  tunnel: ["" w308] -> w297
                  tunnel: [w306 w307] -> w296
                  frame False {
                    # "ignore static sequences"
                  }
                  frame True {
                    # "non-static sequence"
                    n173 = Format Into String(format string="LineRamp(%s_f,%g,%g)", w311, w310, w309) -> (resulting string=w308:string)  [unwired: 2 in, 1 out]
                  }
                }
                n174 = call "Variable.vi"("VariableName"=w299, "InformIgor"=w295, "Sequence"=w296, "SequenceFunction"=w297, "DefaultValue"=w298) -> ("Variable"=w294:refnum<class "Variable.lvclass">)  [unwired: 6 in]
                n175 = call "VariableWrite.vi"("Variable"=w294, "VariableManagerRef in"=w292) -> ("error out"=w291:errorcluster)  [unwired: 8 in, 1 out]
                n176 = call "DisplayMessageAsync.vi"("error in (no error)"=w291) -> ()  [unwired: 11 in]
              }
              n177 = To Unsigned Long Integer(number=w283) -> (unsigned 32bit integer=w281:u32)
              n178 = call "SequenceIndex.vi"("Steps"=w281, "SequenceIndexName"=w282) -> ("SequenceIndex"=w279:refnum<class "SequenceIndex.lvclass">)  [unwired: 9 in]
              n179 = call "SequenceIndexWrite.vi"("SequenceIndex"=w279, "VariableManagerRef in"=w276) -> ("error out"=w277:errorcluster, "VariableManagerRef out"=w278:refnum<vi>)  [unwired: 8 in]
              n180 = call "DisplayMessageAsync.vi"("error in (no error)"=w277) -> ()  [unwired: 11 in]
            }
            frame #1 {
              n181 = call "VMExport.vi"("VariableManagerRef in"=w314) -> ("VariableManagerExportCopy"=w313:refnum<class "VariableManager.lvclass">)  [unwired: 8 in, 2 out]
            }
          }
          n182 = property on="Select Layout" class="Ring (strict)"() -> ("Value"=w269:i32, "StringsAndValues[]"=w268:T3)  [unwired: 2 in, 2 out]
          n183 = local read "User defined functions"() -> (w267:string)
          n184 = local read "Version"() -> (w271:string)
          n185 = local read "Devices"() -> (w270:refnum<class "Device.lvclass">[])
          n186 = Bundle By Name(cluster=T2 {"Version"="", "Devices"=[], "Select Layout"=0, "Layout:Strings And Values []"=[], "User defined functions"="", "VariableManager"=refnum} ("Save Cluster"), "Version"=w271, "Devices"=w270, "Select Layout"=w269, "Layout:Strings And Values []"=w268, "User defined functions"=w267, "VariableManager"=w274) -> (→"Save Cluster":T2)
        }
      }
    }
    frame Error {
    }
  }
  "error out" <- w10
